vi "Set XML Ref.vi"(10 "XML Ref":refnum<k20>, 11 "Project XML Editor in":refnum<class "Project XML Editor.lvclass">) -> (3 "Project XML Editor out":refnum<class "Project XML Editor.lvclass">)   [LabVIEW 2019, in "Project XML Editor.lvclass"]
uses:
  Project XML Editor.lvclass
  Project XML Editor.lvclass/Project XML Editor.ctl
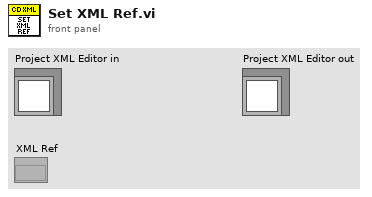
[diagram p1: front panel]
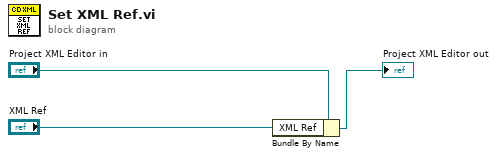
[diagram p0: block diagram]
diagram:
  n1 = Bundle By Name(cluster="Project XML Editor in", "XML Ref"="XML Ref") -> (→"Project XML Editor out":refnum<class "Project XML Editor.lvclass">)
